vi "FPGA Read T2H FIFO Address by Name.vi"(8 "error in (no error)":errorcluster, 9 "Name":string, 10 "Data Type":T1, 11 "FPGA Interface Base in":refnum<class "FPGA Interface Base.lvclass">) -> (0 "error out":errorcluster, 1 "Found?":bool, 2 "Address":u32, 3 "FPGA Interface Base out":refnum<class "FPGA Interface Base.lvclass">)   [LabVIEW 2010, in "FPGA Interface Base.lvclass"]
uses:
  <userlib>/_FPGA Interface Advanced Tools/FPGA Interface Base/FPGA Interface Base.lvclass
  <vilib>/rvi/DataTransferAndStorage/Container/Common/niFpgaDataTypeControl.ctl
  <userlib>/_FPGA Interface Advanced Tools/FPGA Interface Base/FPGA Interface Base.lvclass/FPGA Interface Base.ctl
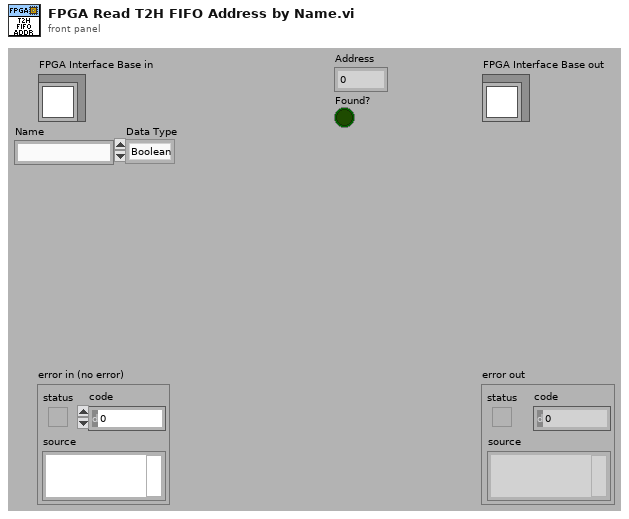
[diagram p1: front panel]
types:
  T1 = typedef "niFpgaDataTypeControl.ctl" = enum32{"Boolean", "I8", "I16", "I32", "I64", "U8", "U16", "U32", "U64", "FXP", "CustomControl"}
  T2 = typedef "FPGA Interface Base.lvclass/FPGA Session.ctl" = refnum<data-value>
  T3 = typedef "FPGA Interface Base.lvclass/FPGA Session Data.ctl" = cluster{"Session Out":u32, "Indicator Scalars":T4, "Indicator Arrays":T6, "Control Scalars":T4, "Control Arrays":T6, "TargetToHost FIFO Channels":T8, "HostToTarget FIFO Channels":T8, "All FIFOs":T9[], "IRQ Context Queue":refnum<queue>}
  T4 = typedef "FPGA Bitfile Utility.lvlib/Scalar Register Set.ctl" = cluster{"Boolean":T5[], "I8":T5[], "I16":T5[], "I32":T5[], "I64":T5[], "U8":T5[], "U16":T5[], "U32":T5[], "U64":T5[]}
  T5 = typedef "FPGA Bitfile Utility.lvlib/Scalar Register.ctl" = cluster{"Address":u32, "Name":string}
  T6 = typedef "FPGA Bitfile Utility.lvlib/Array Register Set.ctl" = cluster{"Boolean":T7[], "I8":T7[], "I16":T7[], "I32":T7[], "I64":T7[], "U8":T7[], "U16":T7[], "U32":T7[], "U64":T7[]}
  T7 = typedef "FPGA Bitfile Utility.lvlib/Array Register.ctl" = cluster{"Address":u32, "Num Elements":u32, "Name":string}
  T8 = typedef "FPGA Bitfile Utility.lvlib/FIFO Channel Set.ctl" = cluster{"Boolean":T9[], "I8":T9[], "I16":T9[], "I32":T9[], "I64":T9[], "U8":T9[], "U16":T9[], "U32":T9[], "U64":T9[]}
  T9 = typedef "FPGA Bitfile Utility.lvlib/FIFO Channel.ctl" = cluster{"Physical Channel":u32, "Name":string}
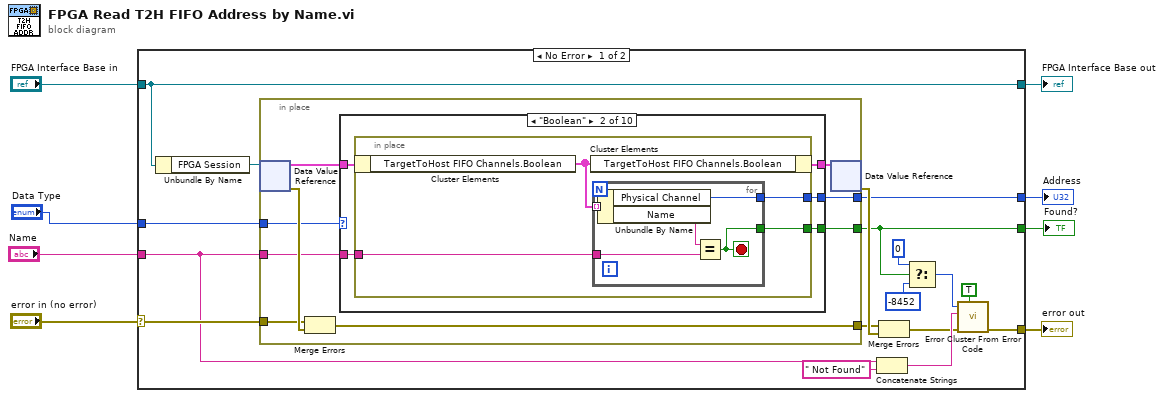
[diagram p0: block diagram]
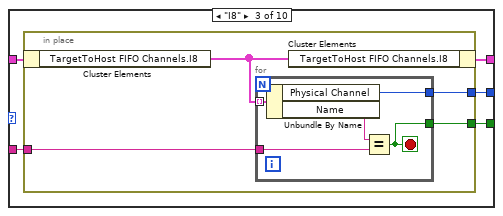
[diagram p3: hidden frame]
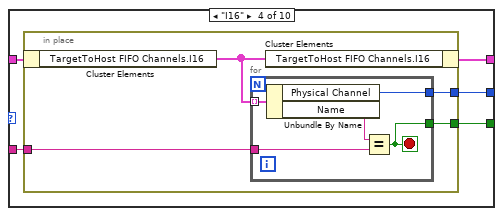
[diagram p4: hidden frame]
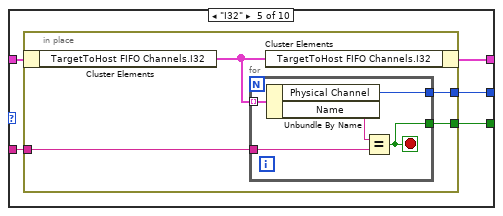
[diagram p5: hidden frame]
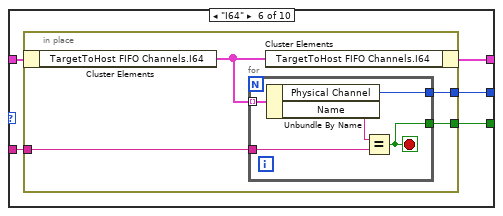
[diagram p6: hidden frame]
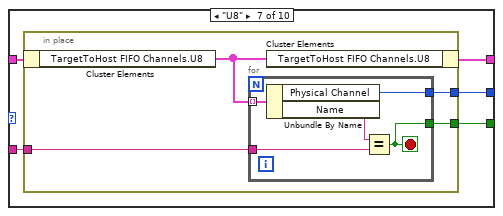
[diagram p7: hidden frame]
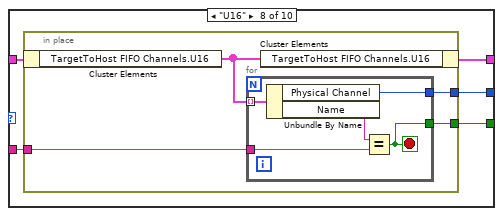
[diagram p8: hidden frame]
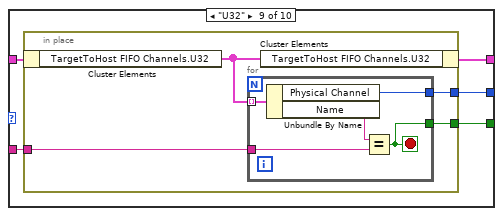
[diagram p9: hidden frame]
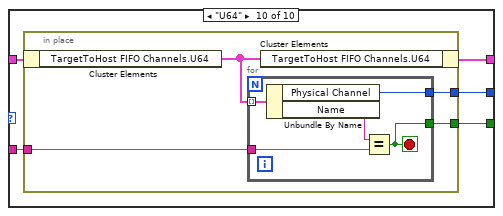
[diagram p10: hidden frame]
diagram:
  n1 = case shown="No Error" "error in (no error)" {
    selector: "error in (no error)" -> [w22 w162]
    tunnel: [w12 w162] -> w7
    tunnel: [w20 w163] -> w5
    tunnel: "FPGA Interface Base in" -> [w20 w163]
    tunnel: [w23 _] -> w4
    tunnel: [w10 _] -> w3
    tunnel: "Name" -> [w9 _]
    tunnel: "Data Type" -> [w21 _]
    frame No Error {
      n2 = Unbundle By Name(w20) -> ("FPGA Session"=w19:T2)
      n3 = in-place {
        in-place-border: w9 -> [w31]
        in-place-border: [w30] -> w23
        in-place-border: [w29] -> w10
        in-place-border: [w28] -> w24
        in-place-border: w22 -> [w27]
        in-place-border: w21 -> [w26]
        n4 = in-place-dvr #1(w19) -> (w33:T3, w34:errorcluster)
        n5 = Merge Errors(w27, w34) -> (w28:errorcluster)
        n6 = case shown="\"Boolean\"" w26 {
          tunnel: w33 -> [w35 w40 w54 w68 w82 w96 w110 w124 w138 w152]
          tunnel: [w35 w39 w53 w67 w81 w95 w109 w123 w137 w151] -> w32
          tunnel: w31 -> [_ w38 w52 w66 w80 w94 w108 w122 w136 w150]
          tunnel: [_ w37 w51 w65 w79 w93 w107 w121 w135 w149] -> w30
          tunnel: [_ w36 w50 w64 w78 w92 w106 w120 w134 w148] -> w29
          frame Default {
          }
          frame "Boolean" {
            n7 = in-place {
              in-place-border: w38 -> [w43]
              in-place-border: [w42] -> w37
              in-place-border: [w41] -> w36
              n8 = in-place-cluster #2(w40) -> ("TargetToHost FIFO Channels.Boolean"=w44:T9[])
              n9 = in-place-cluster #2("TargetToHost FIFO Channels.Boolean"=w44) -> (w39:T3)
              n10 = for {
                tunnel: w44 -> [w49] mode=indexing
                tunnel: [w47] -> w42
                tunnel: [w46] -> w41
                tunnel: w43 -> [w45]
                stop <- w46 stop-if-true
                n11 = Unbundle By Name(w49) -> ("Physical Channel"=w47:u32, "Name"=w48:string)
                n12 = Equal?(x=w48, y=w45) -> (x = y?=w46:bool)
              }
            }
          }
          frame "I8" {
            n13 = in-place {
              in-place-border: w52 -> [w57]
              in-place-border: [w56] -> w51
              in-place-border: [w55] -> w50
              n14 = in-place-cluster #3(w54) -> ("TargetToHost FIFO Channels.I8"=w58:T9[])
              n15 = for {
                tunnel: w58 -> [w63] mode=indexing
                tunnel: [w61] -> w56
                tunnel: [w60] -> w55
                tunnel: w57 -> [w59]
                stop <- w60 stop-if-true
                n16 = Unbundle By Name(w63) -> ("Physical Channel"=w61:u32, "Name"=w62:string)
                n17 = Equal?(x=w62, y=w59) -> (x = y?=w60:bool)
              }
              n18 = in-place-cluster #3("TargetToHost FIFO Channels.I8"=w58) -> (w53:T3)
            }
          }
          frame "I16" {
            n19 = in-place {
              in-place-border: w66 -> [w71]
              in-place-border: [w70] -> w65
              in-place-border: [w69] -> w64
              n20 = in-place-cluster #4(w68) -> ("TargetToHost FIFO Channels.I16"=w72:T9[])
              n21 = for {
                tunnel: w72 -> [w77] mode=indexing
                tunnel: [w75] -> w70
                tunnel: [w74] -> w69
                tunnel: w71 -> [w73]
                stop <- w74 stop-if-true
                n22 = Unbundle By Name(w77) -> ("Physical Channel"=w75:u32, "Name"=w76:string)
                n23 = Equal?(x=w76, y=w73) -> (x = y?=w74:bool)
              }
              n24 = in-place-cluster #4("TargetToHost FIFO Channels.I16"=w72) -> (w67:T3)
            }
          }
          frame "I32" {
            n25 = in-place {
              in-place-border: w80 -> [w85]
              in-place-border: [w84] -> w79
              in-place-border: [w83] -> w78
              n26 = in-place-cluster #5(w82) -> ("TargetToHost FIFO Channels.I32"=w86:T9[])
              n27 = for {
                tunnel: w86 -> [w91] mode=indexing
                tunnel: [w89] -> w84
                tunnel: [w88] -> w83
                tunnel: w85 -> [w87]
                stop <- w88 stop-if-true
                n28 = Unbundle By Name(w91) -> ("Physical Channel"=w89:u32, "Name"=w90:string)
                n29 = Equal?(x=w90, y=w87) -> (x = y?=w88:bool)
              }
              n30 = in-place-cluster #5("TargetToHost FIFO Channels.I32"=w86) -> (w81:T3)
            }
          }
          frame "I64" {
            n31 = in-place {
              in-place-border: w94 -> [w99]
              in-place-border: [w98] -> w93
              in-place-border: [w97] -> w92
              n32 = in-place-cluster #6(w96) -> ("TargetToHost FIFO Channels.I64"=w100:T9[])
              n33 = for {
                tunnel: w100 -> [w105] mode=indexing
                tunnel: [w103] -> w98
                tunnel: [w102] -> w97
                tunnel: w99 -> [w101]
                stop <- w102 stop-if-true
                n34 = Unbundle By Name(w105) -> ("Physical Channel"=w103:u32, "Name"=w104:string)
                n35 = Equal?(x=w104, y=w101) -> (x = y?=w102:bool)
              }
              n36 = in-place-cluster #6("TargetToHost FIFO Channels.I64"=w100) -> (w95:T3)
            }
          }
          frame "U8" {
            n37 = in-place {
              in-place-border: w108 -> [w113]
              in-place-border: [w112] -> w107
              in-place-border: [w111] -> w106
              n38 = in-place-cluster #7(w110) -> ("TargetToHost FIFO Channels.U8"=w114:T9[])
              n39 = for {
                tunnel: w114 -> [w119] mode=indexing
                tunnel: [w117] -> w112
                tunnel: [w116] -> w111
                tunnel: w113 -> [w115]
                stop <- w116 stop-if-true
                n40 = Unbundle By Name(w119) -> ("Physical Channel"=w117:u32, "Name"=w118:string)
                n41 = Equal?(x=w118, y=w115) -> (x = y?=w116:bool)
              }
              n42 = in-place-cluster #7("TargetToHost FIFO Channels.U8"=w114) -> (w109:T3)
            }
          }
          frame "U16" {
            n43 = in-place {
              in-place-border: w122 -> [w127]
              in-place-border: [w126] -> w121
              in-place-border: [w125] -> w120
              n44 = in-place-cluster #8(w124) -> ("TargetToHost FIFO Channels.U16"=w128:T9[])
              n45 = for {
                tunnel: w128 -> [w133] mode=indexing
                tunnel: [w131] -> w126
                tunnel: [w130] -> w125
                tunnel: w127 -> [w129]
                stop <- w130 stop-if-true
                n46 = Unbundle By Name(w133) -> ("Physical Channel"=w131:u32, "Name"=w132:string)
                n47 = Equal?(x=w132, y=w129) -> (x = y?=w130:bool)
              }
              n48 = in-place-cluster #8("TargetToHost FIFO Channels.U16"=w128) -> (w123:T3)
            }
          }
          frame "U32" {
            n49 = in-place {
              in-place-border: w136 -> [w141]
              in-place-border: [w140] -> w135
              in-place-border: [w139] -> w134
              n50 = in-place-cluster #9(w138) -> ("TargetToHost FIFO Channels.U32"=w142:T9[])
              n51 = for {
                tunnel: w142 -> [w147] mode=indexing
                tunnel: [w145] -> w140
                tunnel: [w144] -> w139
                tunnel: w141 -> [w143]
                stop <- w144 stop-if-true
                n52 = Unbundle By Name(w147) -> ("Physical Channel"=w145:u32, "Name"=w146:string)
                n53 = Equal?(x=w146, y=w143) -> (x = y?=w144:bool)
              }
              n54 = in-place-cluster #9("TargetToHost FIFO Channels.U32"=w142) -> (w137:T3)
            }
          }
          frame "U64" {
            n55 = in-place {
              in-place-border: w150 -> [w155]
              in-place-border: [w154] -> w149
              in-place-border: [w153] -> w148
              n56 = in-place-cluster #10(w152) -> ("TargetToHost FIFO Channels.U64"=w156:T9[])
              n57 = for {
                tunnel: w156 -> [w161] mode=indexing
                tunnel: [w159] -> w154
                tunnel: [w158] -> w153
                tunnel: w155 -> [w157]
                stop <- w158 stop-if-true
                n58 = Unbundle By Name(w161) -> ("Physical Channel"=w159:u32, "Name"=w160:string)
                n59 = Equal?(x=w160, y=w157) -> (x = y?=w158:bool)
              }
              n60 = in-place-cluster #10("TargetToHost FIFO Channels.U64"=w156) -> (w151:T3)
            }
          }
        }
        n61 = in-place-dvr #1(w32) -> (w25:errorcluster)  [unwired: 1 out]
      }
      n62 = Concatenate Strings(w9, " Not Found" ("string")) -> (w18:string)
      n63 = Merge Errors(w24, w25) -> (w11:errorcluster)
      n64 = Select(t=0, s=w10, f=-8452 ("error code (0)")) -> (s? t:f=w13:i32)
      n65 = call <vilib>:"Error Cluster From Error Code.vi"("show call chain? (False)"=TRUE, "error in (no error)"=w11, "error message (\"\")"=w18, "error code (0)"=w13) -> ("error out"=w12:errorcluster)  [unwired: 5 in]
    }
    frame Error {
    }
  }
  "error out" <- w7
  "FPGA Interface Base out" <- w5
  "Address" <- w4
  "Found?" <- w3
